vi "Configure Modulation (Custom).vi"(0 "VISA resource name":refnum<visa-resource-name>, 1 "Enable Custom Modulation (T:Enable)":bool=TRUE, 2 "MSK Phase Deviation (90 deg)":dbl=90.0, 3 "FSK Frequency Deviation (400 Hz)":dbl=400.0, 5 "Standard (0: None)":u16(ring) items=["None", "APCO 25 w/C4FM", "APCO 25 w/CQPSK", "Bluetooth", "CDPD"], 7 "Modulation Type (6: pi/4 DQPSK)":u16(ring)=6 items=["BPSK", "QPSK", "IS-95 QPSK", "Gray Coded QPSK", "OQPSK", "IS-95 OQPSK", "pi/4 DQPSK", "8PSK", "16PSK", "D8PSK", "MSK", "2-Lvl FSK", "4-Lvl FSK", "8-Lvl FSK", "16-Lvl FSK", "C4FM", "4QAM", "16QAM", "32QAM", "64QAM", "128QAM", "256QAM", "User I/Q", "User FSK"], 9 "File Name (\"\")":string, 11 "error in (no error)":errorcluster, 12 "Symbol Rate (24.3 kbps)":dbl=24300.0, 13 "I/Q Scaling (70 percent)":dbl=70.0, 14 "Phase Polarity (0: Normal)":u16(ring) items=["Normal", "Inverted"]) -> (4 "VISA resource name out":refnum<visa-resource-name>, 15 "error out":errorcluster)   [LabVIEW 2011, in "Agilent PSG MXG Series.lvlib"]
doc: "Configures the state, type, standard, phase polarity, I/Q scaling value and symbol rate for the custom modulation.\n\n<B>Notes:</B>\n(1) This VI is valid only in E8267C, E8267D.\n\n(2) For E8267C, this VI is valid only when the instrument installs <B>Option 002</B> (Internal baseband generator) or <B>Option 602</B> (Digital bus baseband generator).\n\n(3) For E8267D, this VI is valid only when the instrument installs <B>Option 601</B> or <B>Option 602</B> (Internal baseband generator)."
uses:
  Agilent PSG MXG Series.lvlib
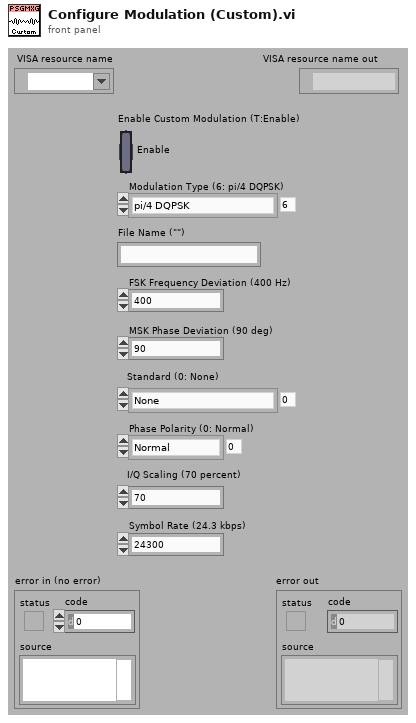
[diagram p1: front panel]
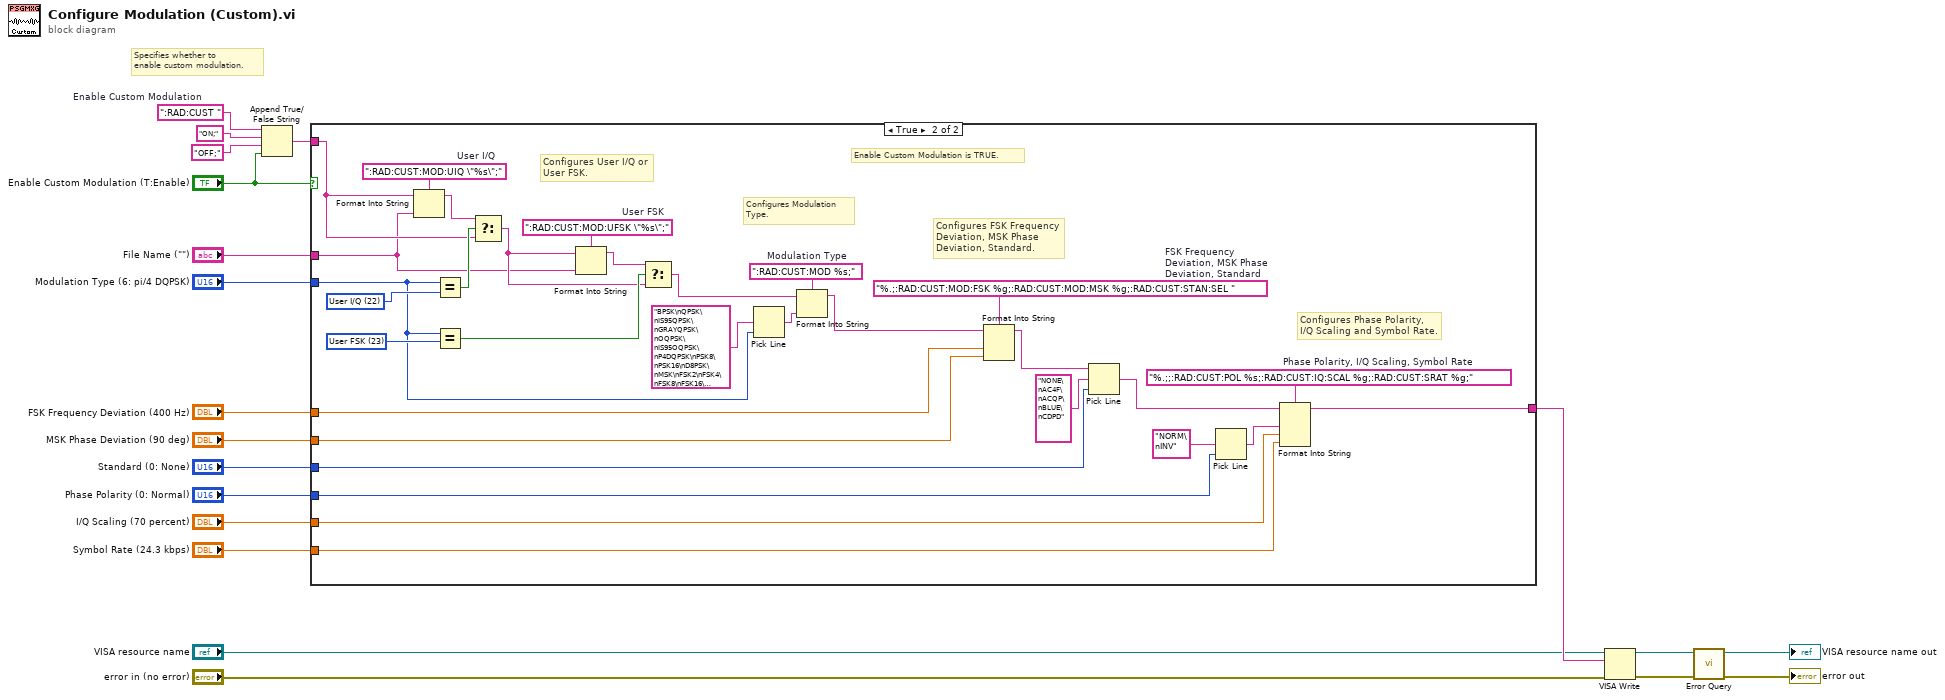
[diagram p0: block diagram]
diagram:
  w20 = ":RAD:CUST "  # Enable Custom Modulation
  # "Specifies whether to\nenable custom modulation."
  n1 = Append True/False String(1:"Enable Custom Modulation (T:Enable)", 2:"OFF;" ("false string"), 3:"ON;" ("true string"), 4:w20) -> (0:w16:string)
  n2 = case shown="True" "Enable Custom Modulation (T:Enable)" {
    tunnel: w16 -> [w21 w30]
    tunnel: "Modulation Type (6: pi/4 DQPSK)" -> [_ w23]
    tunnel: "File Name (\"\")" -> [_ w28]
    tunnel: "FSK Frequency Deviation (400 Hz)" -> [_ w43]
    tunnel: "MSK Phase Deviation (90 deg)" -> [_ w42]
    tunnel: "Standard (0: None)" -> [_ w39]
    tunnel: "Phase Polarity (0: Normal)" -> [_ w34]
    tunnel: "I/Q Scaling (70 percent)" -> [_ w33]
    tunnel: "Symbol Rate (24.3 kbps)" -> [_ w32]
    tunnel: [w21 w31] -> w7
    frame False {
      # "Enable Custom Modulation\nis FALSE."
    }
    frame True {
      w25 = ":RAD:CUST:MOD %s;"  # Modulation Type
      w37 = "%.;;:RAD:CUST:POL %s;:RAD:CUST:IQ:SCAL %g;:RAD:CUST:SRAT %g;"  # Phase Polarity, I/Q Scaling, Symbol Rate
      w44 = "%.;:RAD:CUST:MOD:FSK %g;:RAD:CUST:MOD:MSK %g;:RAD:CUST:STAN:SEL "  # FSK Frequency Deviation, MSK Phase Deviation, Standard
      w47 = ":RAD:CUST:MOD:UFSK \"%s\";"  # User FSK
      w48 = u16 23 items=["BPSK", "QPSK", "IS-95 QPSK", "Gray Coded QPSK", "OQPSK", "IS-95 OQPSK", "pi/4 DQPSK", "8PSK", "16PSK", "D8PSK", "MSK", "2-Lvl FSK", "4-Lvl FSK", "8-Lvl FSK", "16-Lvl FSK", "C4FM", "4QAM", "16QAM", "32QAM", "64QAM", "128QAM", "256QAM", "User I/Q", "User FSK"] ("Modulation Type (6: pi/4 DQPSK)")
      w52 = ":RAD:CUST:MOD:UIQ \"%s\";"  # User I/Q
      w51 = u16 22 items=["BPSK", "QPSK", "IS-95 QPSK", "Gray Coded QPSK", "OQPSK", "IS-95 OQPSK", "pi/4 DQPSK", "8PSK", "16PSK", "D8PSK", "MSK", "2-Lvl FSK", "4-Lvl FSK", "8-Lvl FSK", "16-Lvl FSK", "C4FM", "4QAM", "16QAM", "32QAM", "64QAM", "128QAM", "256QAM", "User I/Q", "User FSK"] ("Modulation Type (6: pi/4 DQPSK)")
      # "Configures Phase Polarity,\nI/Q Scaling and Symbol Rate."
      # "Configures FSK Frequency\nDeviation, MSK Phase\nDeviation, Standard."
      # "Configures Modulation\nType."
      # "Configures User I/Q or\nUser FSK."
      # "Enable Custom Modulation is TRUE."
      n3 = Format Into String(format string=w52, initial string=w30, w28) -> (resulting string=w49:string)  [unwired: 1 in, 1 out]
      n4 = Equal?(x=w23, y=w51) -> (x = y?=w50:bool)
      n5 = Equal?(x=w23, y=w48) -> (x = y?=w46:bool)
      n6 = Select(t=w49, s=w50, f=w30) -> (s? t:f=w45:string)
      n7 = Format Into String(format string=w47, initial string=w45, w28) -> (resulting string=w29:string)  [unwired: 1 in, 1 out]
      n8 = Select(t=w29, s=w46, f=w45) -> (s? t:f=w26:string)
      n9 = Pick Line(multi-line string="BPSK\nQPSK\nIS95QPSK\nGRAYQPSK\nOQPSK\nIS95OQPSK\nP4DQPSK\nPSK8\nPSK16\nD8PSK\nMSK\nFSK2\nFSK4\nFSK8\nFSK16\nC4FM\nQAM4\nQAM16\nQAM32\nQAM64\nQAM128\nQAM256\nUIQ\nUFSK", line index=w23) -> (output string=w27:string)  [unwired: 1 in]
      n10 = Format Into String(format string=w25, initial string=w26, w27) -> (resulting string=w22:string)  [unwired: 1 in, 1 out]
      n11 = Format Into String(format string=w44, initial string=w22, w43, w42) -> (resulting string=w41:string)  [unwired: 1 in, 1 out]
      n12 = Pick Line(string ("")=w41, multi-line string="NONE\nAC4F\nACQP\nBLUE\nCDPD", line index=w39) -> (output string=w38:string)
      n13 = Pick Line(multi-line string="NORM\nINV", line index=w34) -> (output string=w36:string)  [unwired: 1 in]
      n14 = Format Into String(format string=w37, initial string=w38, w36, w33, w32) -> (resulting string=w31:string)  [unwired: 1 in, 1 out]
    }
  }
  n15 = VISA Write(VISA resource name="VISA resource name", write buffer=w7, error in (no error)="error in (no error)") -> (VISA resource name out=w6:refnum<visa-resource-name>, error out=w5:errorcluster)  [unwired: 1 out]
  n16 = call "Error Query.vi"("error in (no error)"=w5, "VISA resource name"=w6) -> ("error out"=→"error out":errorcluster, "VISA resource name out"=→"VISA resource name out":refnum<visa-resource-name>)  [unwired: 6 in, 2 out]
